vi "test Set Odd Parity by Index.vi"(8 "error in (no error)":errorcluster, 11 "TestCase in":refnum<class "Parity.lvclass">) -> (0 "error out":errorcluster, 3 "TestCase out":refnum<class "Parity.lvclass">)   [LabVIEW 2027, in "Parity.lvclass"]
uses:
  Parity.lvclass
  Source/Parity.ctl
  b79821fd-afdc-4fd3-a910-5010e2989e8e.vi
  C:/Program Files/National Instruments/LabVIEW 2027/vi.lib/addons/_JKI Toolkits/VI Tester/TestCase.llb/TestCase.lvclass
  <vilib>/addons/_JKI Toolkits/VI Tester/TestCase.llb/TestCase.lvclass
  Source/Encoding and Decoding.lvlib
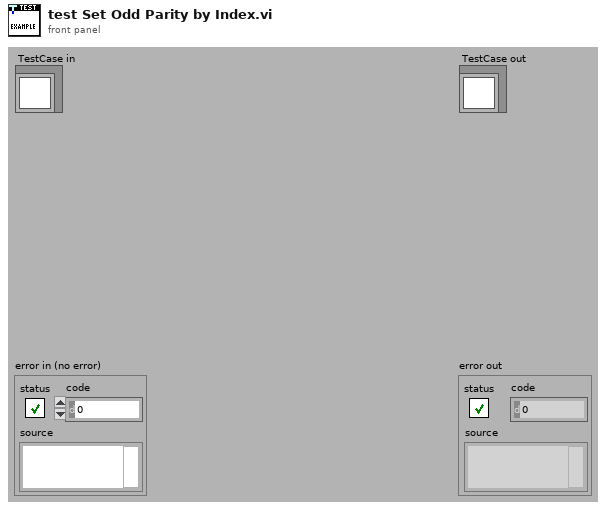
[diagram p1: front panel]
types:
  T1 = typedef "Encoding and Decoding.lvlib/Parity.ctl" = enum16{"Even", "Odd"}
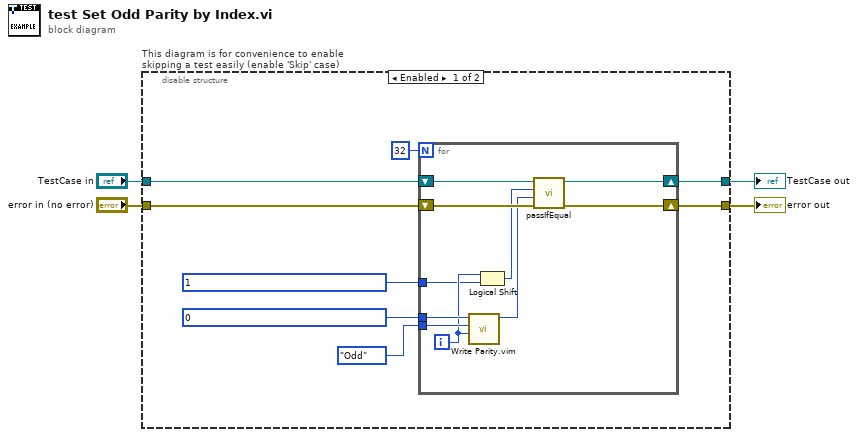
[diagram p0: block diagram]
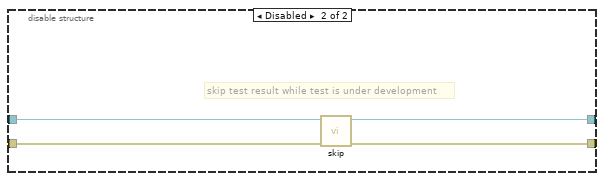
[diagram p2: hidden frame]
diagram:
  n1 = disable-structure "This diagram is for convenience to enable skipping a test easily (enable 'Skip' case)" shown="Enabled" {
    disable-tunnel: "TestCase in" -> [w12 w26]
    disable-tunnel: [w5 w24] -> w1
    disable-tunnel: [w6 w25] -> w3
    disable-tunnel: "error in (no error)" -> [w11 w23]
    frame Enabled {
      n2 = for {
        N: 32 -> [_]
        tunnel: u32 0 ("word in") -> [w20]
        tunnel: Parity."Odd" ("parity") -> [w18]
        tunnel: u32 1 ("word in") -> [w13]
        shift-right: [w17] -> w5
        shift-left: w12 -> [w22]
        shift-right: [w16] -> w6
        shift-left: w11 -> [w21]
        i -> [w15]
        n3 = call "Write Parity.vim"("parity index"=w15, "parity"=w18, "word in"=w20) -> ("word out"=w19:u32)  [unwired: 8 in]
        n4 = Logical Shift(y=w15, x=w13) -> (x << y=w14:u32)
        n5 = call-dynamic "passIfEqual.vi"("error in (no error)"=w21, "y"=w19, "x"=w14, "TestCase in"=w22) -> ("error out"=w16:errorcluster, "TestCase out"=w17:refnum<class "Parity.lvclass">)  [unwired: 6 in]
      }
    }
    frame Disabled {
      # "skip test result while test is under development"
      n6 = call <vilib>:"skip.vi"("error in (no error)"=w23, "TestCase in"=w26) -> ("error out"=w25:errorcluster, "TestCase out"=w24:refnum<class "Parity.lvclass">)  [unwired: 8 in]
    }
  }
  "error out" <- w3
  "TestCase out" <- w1
